vi "Decorate.vi"(10 "Queue":refnum<class "Queue.lvclass">, 11 "TEMPLATE Queue in":refnum<class "TEMPLATE Queue.lvclass">) -> (3 "TEMPLATE Queue out":refnum<class "TEMPLATE Queue.lvclass">)   [LabVIEW 2021, in "_Template.lvlib" / "Templates.lvlib" / "TEMPLATE Queue.lvlib" / "TEMPLATE Queue.lvclass"]
uses:
  TEMPLATE Queue.lvclass
  TEMPLATE Queue.lvclass/TEMPLATE Queue.ctl
  jettl/jettl/Queue/Queue.lvclass
  jettl/Setup Msg Strategy/Setup Msg Strategy.lvlib
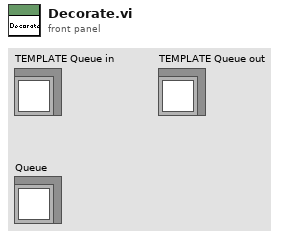
[diagram p1: front panel]
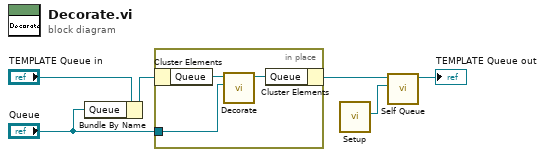
[diagram p0: block diagram]
diagram:
  n1 = Bundle By Name(cluster="TEMPLATE Queue in", "Queue"="Queue") -> (w5:refnum<class "TEMPLATE Queue.lvclass">)
  n2 = in-place {
    in-place-border: "Queue" -> [w7]
    n3 = in-place-cluster #1(w5) -> ("Queue"=w9:refnum<class "Queue.lvclass">)
    n4 = call-dynamic "Decorate.vi"("Queue"=w7, "Queue in"=w9) -> ("Queue out"=w8:refnum<class "Queue.lvclass">)  [unwired: 9 in]
    n5 = in-place-cluster #1("Queue"=w8) -> (w4:refnum<class "TEMPLATE Queue.lvclass">)
  }
  n6 = call "Setup.vi"() -> ("Msg Strategy"=w1:refnum<class "Msg Strategy.lvclass">)  [unwired: 11 in]
  n7 = call-dynamic "Self Queue.vi"("Msg Strategy"=w1, "TEMPLATE Queue in"=w4) -> ("TEMPLATE Queue out"=→"TEMPLATE Queue out":refnum<class "TEMPLATE Queue.lvclass">)  [unwired: 9 in]
